vi "Destroy User Events.vi"(11 "UI Template in":refnum<class "DisplayConsole.lvclass">) -> (3 "UI Template out":refnum<class "DisplayConsole.lvclass">)   [LabVIEW 2025, in "DisplayConsole.lvlib" / "DisplayConsole.lvclass"]
uses:
  DisplayConsole.lvclass
  DisplayConsole.lvclass/DisplayConsole.ctl
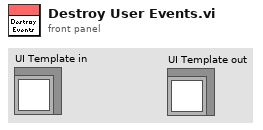
[diagram p1: front panel]
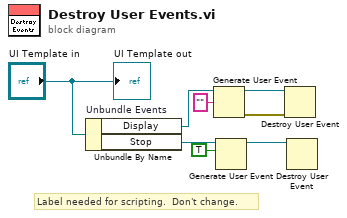
[diagram p0: block diagram]
diagram:
  # "Label needed for scripting.  Don't change."
  n1 = Unbundle By Name "Unbundle Events"("UI Template in") -> ("Display"=w2:refnum<user-event>, "Stop"=w6:refnum<user-event>)
  n2 = Generate User Event(user event=w2, event data cluster="") -> (user event out=w4:refnum<user-event>, error out=w1:errorcluster)  [unwired: 2 in]
  n3 = Generate User Event(user event=w6, event data cluster=TRUE ("event data")) -> (user event out=w7:refnum<user-event>)  [unwired: 2 in, 1 out]
  n4 = Destroy User Event(user event=w4, error in=w1) -> ()  [unwired: 1 out]
  n5 = Destroy User Event(user event=w7) -> ()  [unwired: 1 in, 1 out]
  "UI Template out" <- "UI Template in"
